vi "数据查询_数据查询.vi"() -> ()   [LabVIEW 2016]
uses:
  <vilib>/Utility/miscctls.llb/LVPointTypeDef.ctl
  <vilib>/Utility/miscctls.llb/LVRowAndColumnUnsignedTypeDef.ctl
  <userlib>/_OpenG.lib/array/array.llb/Sort 2D Array (String)__ogtk.vi
  <vilib>/addons/database/_DB Variant To Data/Database Variant To Data.xnode
panel:
  in  "导出":bool
  out "分钟小时":string(combo)="实时数据"
  out "工作类型":string(combo)="全部数据"
  in  "工作模式":string(combo)="全部数据"
  out "连接的字符串":string
  out "选中数据表":string
  in  "查询":bool
  in  "结束日期":string="2020/01/01"
  in  "起始日期":string="2010/01/01"
  out "XY图":cluster{"data":timestamp[], "data":dbl[]}[](graph)
  in  "组合框":string(combo)
  out "数据表":string[][](table)
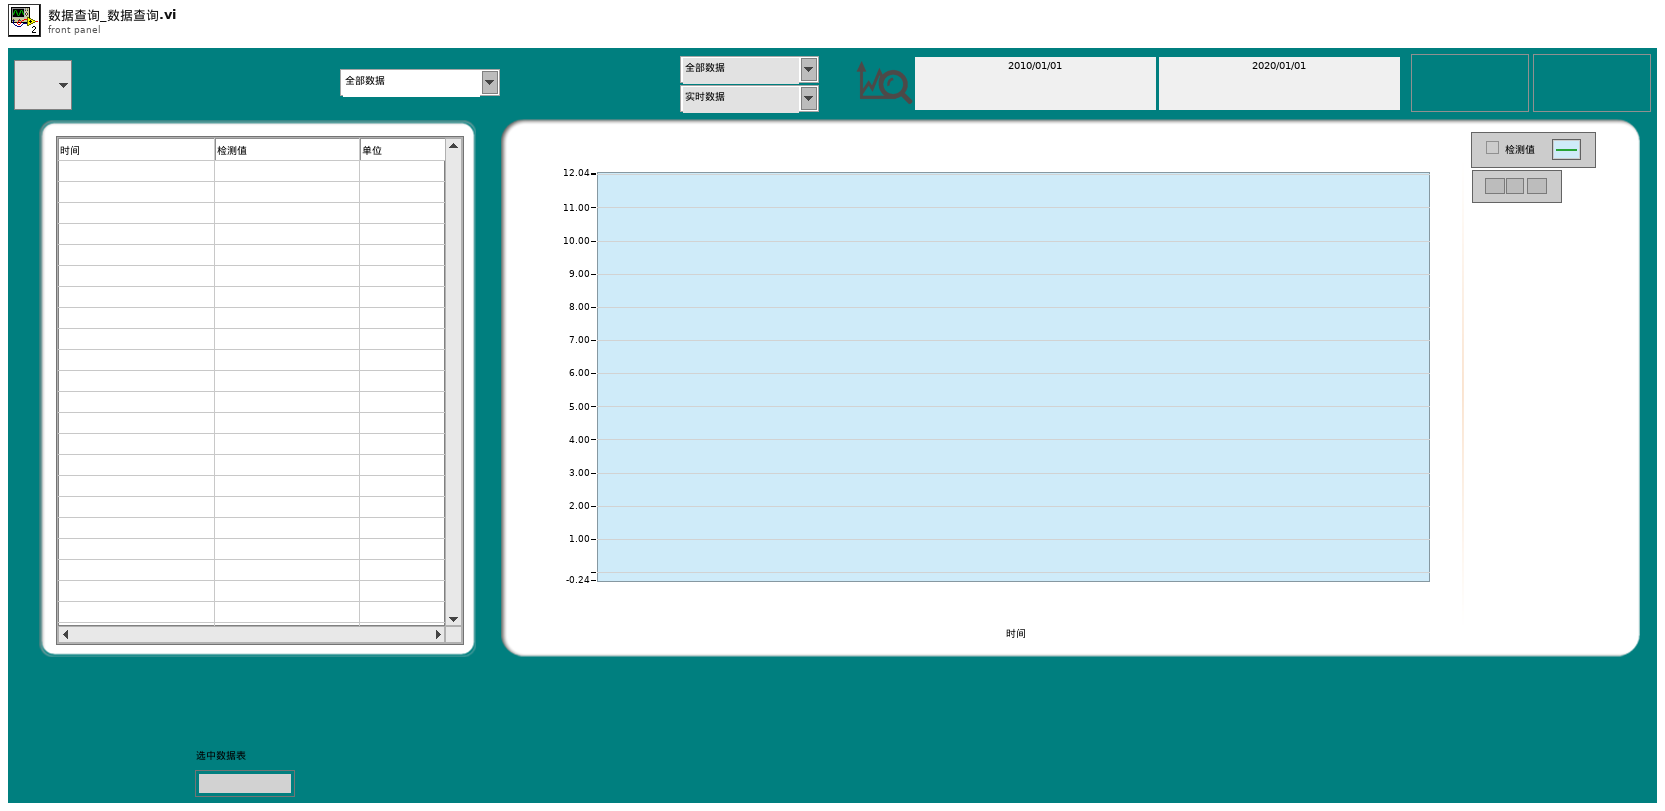
[diagram p1: front panel]
types:
  T1 = typedef "LVPointTypeDef.ctl" = cluster{"Horizontal":i16, "Vertical":i16}
  T2 = enum8{"Enabled", "Disabled", "Disabled and Grayed Out"}
  T3 = typedef "LVRowAndColumnUnsignedTypeDef.ctl" = cluster{"Row":u32, "Column":u32}
  T4 = typedef "LVPoint32TypeDef.ctl" = cluster{"Horizontal":i32, "Vertical":i32}
  T5 = typedef "LVPointDoubleTypeDef.ctl" = cluster{"Cursor X":dbl, "Cursor Y":dbl}
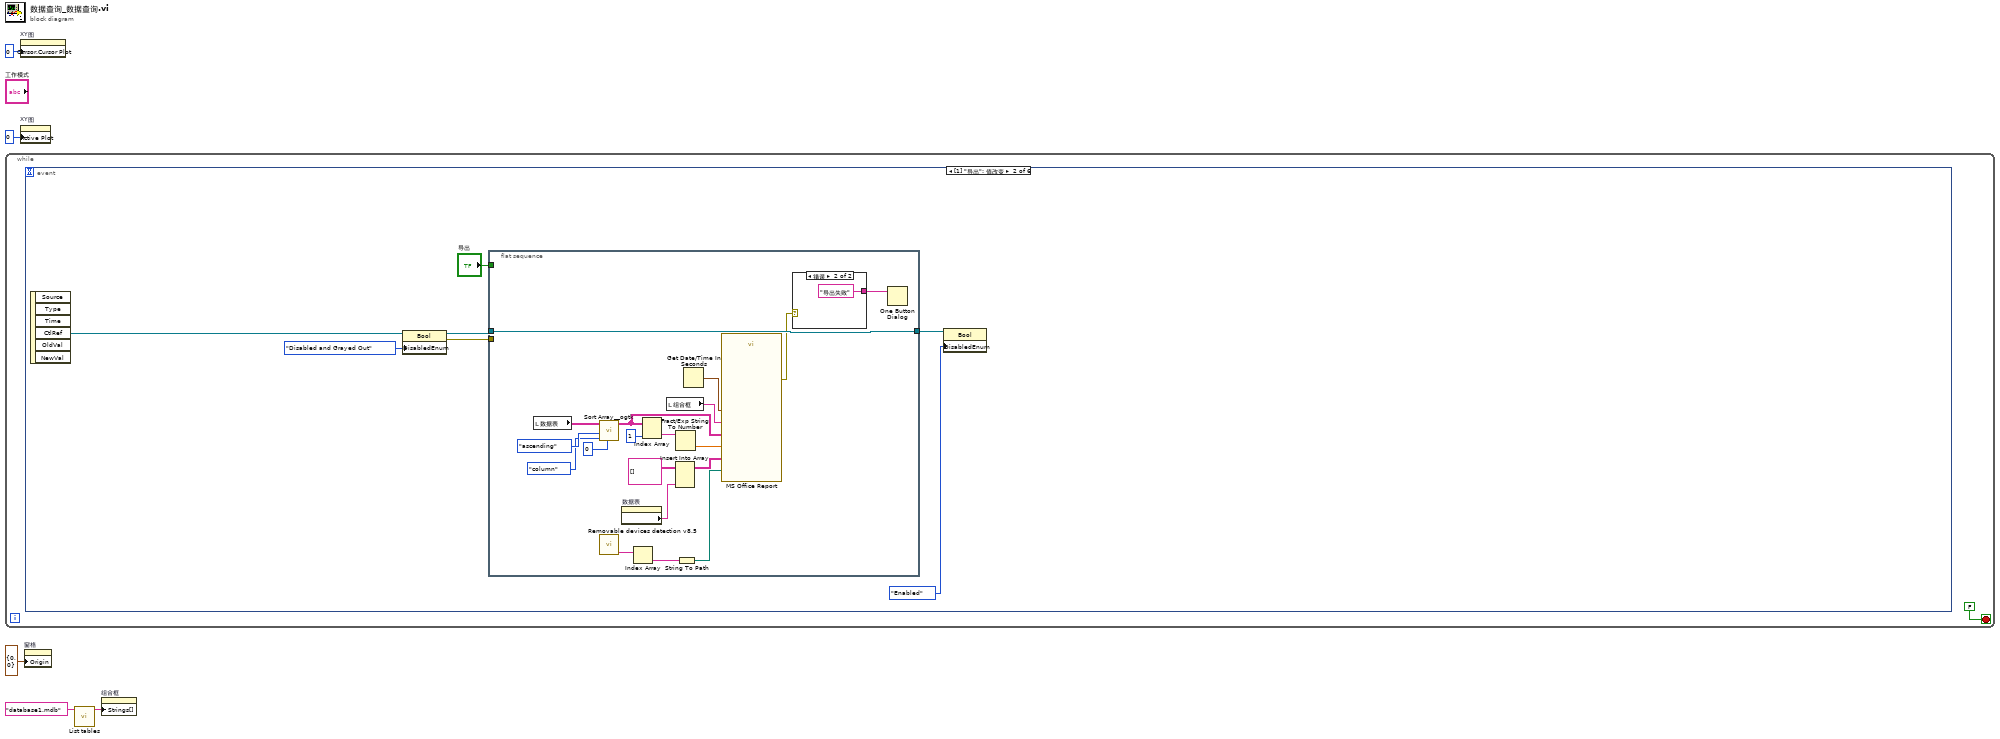
[diagram p0: block diagram]
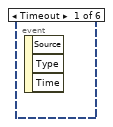
[diagram p2: hidden frame]
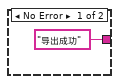
[diagram p3: hidden frame]
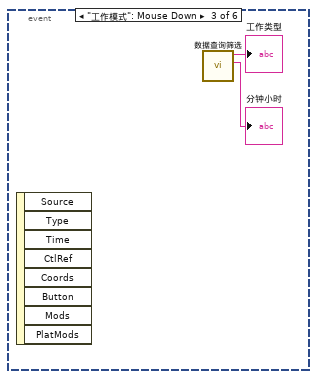
[diagram p4: hidden frame]
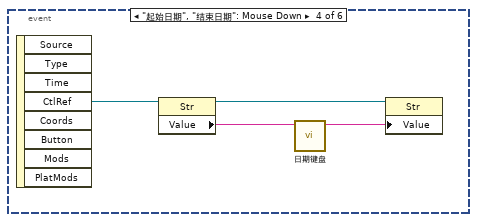
[diagram p5: hidden frame]
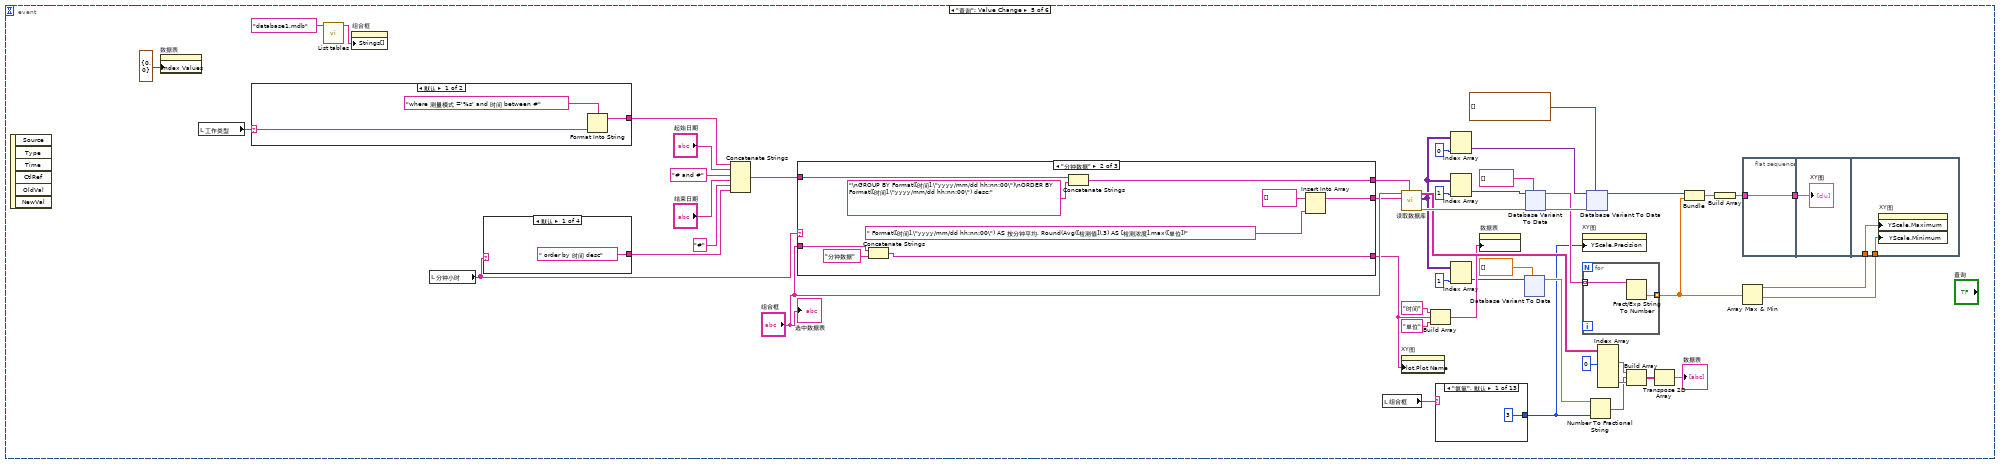
[diagram p6: hidden frame]
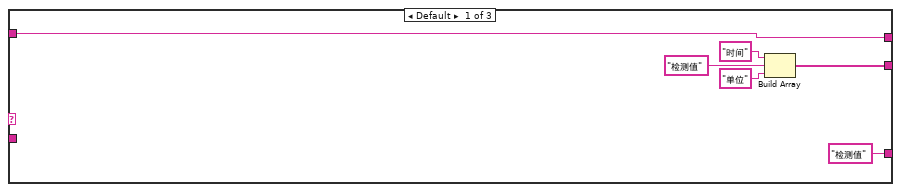
[diagram p7: hidden frame]
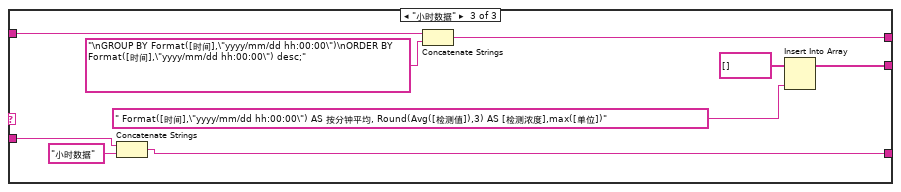
[diagram p8: hidden frame]
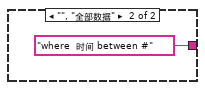
[diagram p12: hidden frame]
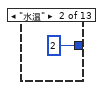
[diagram p13: hidden frame]
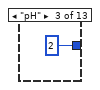
[diagram p14: hidden frame]
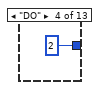
[diagram p15: hidden frame]
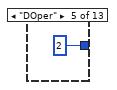
[diagram p16: hidden frame]
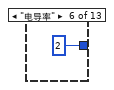
[diagram p17: hidden frame]
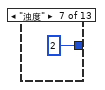
[diagram p18: hidden frame]
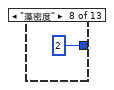
[diagram p19: hidden frame]
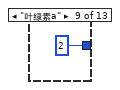
[diagram p20: hidden frame]
diagram:
  n1 = while {
    stop <- FALSE stop-if-true
    n2 = event shown="[1] \"导出\": 值改变" {
      selector: _ -> [_ _ _ _ _ _]
      dyn-events: _ -> [_ _ _ _ _ _]
      timeout: _ -> [_ _ _ _ _ _]
      event Timeout {
        n3 = event-data() -> ()  [unwired: 1 in, 3 out]
      }
      event "导出": Value Change {
        n4 = event-data() -> ("CtlRef"=w13:refnum<vi>)  [unwired: 1 in, 5 out]
        n5 = property class="Bool"(reference=w13, "DisabledEnum"=T2."Disabled and Grayed Out" ("禁用")) -> (reference out=w10:refnum<vi>, error out=w11:errorcluster)  [unwired: 1 in]
        n6 = flat-sequence {
          tunnel: w11 -> [_]
          tunnel: [w22] -> w9
          tunnel: w10 -> [w22]
          tunnel: "导出" -> [_]
          frame #0 {
            n7 = local read "数据表"() -> (w30:string[][])
            n8 = call-poly <userlib>:"Sort Array__ogtk.vi"("Column/Row to Sort By"=u32 0, "Sort By in"=enum16{"row", "column"}."column", "Order"=enum16{"ascending", "descending"}."ascending", "Array in"=w30) -> ("Sorted Array out"=w29:string[][])  [unwired: 4 in, 3 out]
            n9 = call "Removable devices detection v8.5.vi"() -> ("Removable"=w19:string[])  [unwired: 4 out]
            n10 = property on="数据表" class="Tbl (严格)"() -> ("Column Headers[]"=w15:string[])  [unwired: 2 in, 2 out]
            n11 = Index Array(array=w19) -> (element=w18:string)  [unwired: 1 in]
            n12 = Index Array(array=w29, index (col)=1 ("禁用的索引 (列)")) -> (element=w25:string[])  [unwired: 1 in]
            n13 = local read "组合框"() -> (w23:string)
            n14 = Insert Into Array(array=string[][] [], new element=w15) -> (w14:string[][])  [unwired: 2 in]
            n15 = Fract/Exp String To Number(string=w25) -> (number=w24:dbl[])  [unwired: 3 in, 1 out]
            n16 = String To Path(string=w18) -> (path=w17:path)
            n17 = Get Date/Time In Seconds() -> (seconds since 1Jan1904=w32:timestamp)
            n18 = call "MS Office Report"("Path to Save Report"=w17, "导出日期"=w32, "监测参数"=w23, "数据输入"=w29, "图表输入"=w24, "字段定义"=w14) -> ("error out"=w21:errorcluster)  [unwired: 20 in, 1 out]
            n19 = case shown="错误" w21 {
              tunnel: ["导出成功" ("消息") "导出失败" ("消息")] -> w20
              frame No Error {
              }
              frame Error {
              }
            }
            n20 = One Button Dialog(message=w20) -> ()  [unwired: 1 in, 1 out]
          }
        }
        n21 = property class="Bool"(reference=w9, "DisabledEnum"=T2."Enabled" ("禁用")) -> ()  [unwired: 1 in, 2 out]
      }
      event "工作模式": Mouse Down {
        n22 = event-data() -> ()  [unwired: 1 in, 8 out]
        n23 = call "数据查询筛选.vi"() -> ("分钟小时"=→"分钟小时":string, "工作类型"=→"工作类型":string)  [unwired: 10 in]
      }
      event "起始日期", "结束日期": Mouse Down {
        n24 = event-data() -> ("CtlRef"=w40:refnum<vi>)  [unwired: 1 in, 7 out]
        n25 = property class="Str"(reference=w40) -> (reference out=w38:refnum<vi>, "Value"=w39:string)  [unwired: 1 in, 1 out]
        n26 = call "日期键盘.vi"("原值"=w39) -> ("x+y"=w37:string)  [unwired: 10 in]
        n27 = property class="Str"(reference=w38, "Value"=w37) -> ()  [unwired: 1 in, 2 out]
      }
      event "查询": Value Change {
        n28 = event-data() -> ()  [unwired: 1 in, 6 out]
        n29 = property on="数据表" class="Tbl (严格)"("Index Values"=T3 {"Row"=0, "Column"=0} ("索引值")) -> ()  [unwired: 2 in, 2 out]
        n30 = local read "工作类型"() -> (w49:string)
        n31 = case shown="默认" w49 {
          selector: w49 -> [w117 _]
          tunnel: [w115 "where  时间 between #" ("condition")] -> w48
          frame Default {
            n32 = Format Into String(format string="where 测量模式 ='%s' and 时间 between #" ("condition"), w117) -> (resulting string=w115:string)  [unwired: 2 in, 1 out]
          }
          frame "", "全部数据" {
          }
        }
        n33 = call "List tables.vi"("database"="database1.mdb") -> ("tables"=w55:string[])  [unwired: 9 in, 1 out]
        n34 = property on="组合框" class="CmbBox"("Strings[]"=w55) -> ()  [unwired: 2 in, 2 out]
        n35 = local read "分钟小时"() -> (w45:string)
        n36 = case shown="默认" w45 {
          tunnel: [" order by 时间 desc" ("字符串") _ _ _] -> w47
          frame Default {
          }
          frame "分钟数据" {
          }
          frame "小时数据" {
          }
          frame "真" {
          }
        }
        n37 = Concatenate Strings(w48, "起始日期", "# and #" ("condition"), "结束日期", "#" ("condition"), w47) -> (w46:string)
        n38 = case shown="\"分钟数据\"" w45 {
          tunnel: [w91 w103 w108] -> w42
          tunnel: w46 -> [w95 w101 w110]
          tunnel: [w95 w100 w109] -> w44
          tunnel: ["检测值" w96 w105] -> w41
          tunnel: "组合框" -> [_ w97 w107]
          frame Default {
            n39 = Build Array("时间", "检测值", "单位" ("元素")) -> (w91:string[])
          }
          frame "分钟数据" {
            n40 = Concatenate Strings(w97, "分钟数据" ("字符串")) -> (w96:string)
            n41 = Concatenate Strings(w101, "\nGROUP BY Format([时间],\"yyyy/mm/dd hh:nn:00\")\nORDER BY Format([时间],\"yyyy/mm/dd hh:nn:00\") desc;" ("字符串")) -> (w100:string)
            n42 = Insert Into Array(array=string[] [] ("显示项"), new element=" Format([时间],\"yyyy/mm/dd hh:nn:00\") AS 按分钟平均, Round(Avg([检测值]),3) AS [检测浓度],max([单位])" ("新元素/子数组")) -> (w103:string[])  [unwired: 1 in]
          }
          frame "小时数据" {
            n43 = Concatenate Strings(w107, "小时数据" ("字符串")) -> (w105:string)
            n44 = Concatenate Strings(w110, "\nGROUP BY Format([时间],\"yyyy/mm/dd hh:00:00\")\nORDER BY Format([时间],\"yyyy/mm/dd hh:00:00\") desc;" ("字符串")) -> (w109:string)
            n45 = Insert Into Array(array=string[] [] ("显示项"), new element=" Format([时间],\"yyyy/mm/dd hh:00:00\") AS 按分钟平均, Round(Avg([检测值]),3) AS [检测浓度],max([单位])" ("新元素/子数组")) -> (w108:string[])  [unwired: 1 in]
          }
        }
        n46 = local read "组合框"() -> (w56:string)
        n47 = call "读取数据库.vi"("condition"=w44, "显示项"=w42, "组合框"="组合框") -> ("error out"=w80:errorcluster, "data"=w63:variant[][], "表格"=w73:string[][])  [unwired: 5 in, 1 out]
        n48 = property on="XY图" class="XYGraph (严格)"("Plot.Plot Name"=w41) -> ()  [unwired: 2 in, 2 out]
        n49 = Build Array("时间", w41, "单位" ("元素")) -> (w67:string[])
        n50 = case shown="\"氨氮\", 默认" w56 {
          tunnel: [i16 3 ("精度(6)") i16 2 ("精度(6)") i16 2 ("精度(6)") i16 2 ("精度(6)") i16 2 ("精度(6)") i16 2 ("精度(6)") i16 2 ("精度(6)") i16 2 ("精度(6)") i16 2 ("精度(6)") i16 3 ("精度(6)") i16 3 ("精度(6)") i16 2 ("精度(6)") i16 2 ("精度(6)")] -> w50
          frame "氨氮", Default {
          }
          frame "水温" {
          }
          frame "pH" {
          }
          frame "DO" {
          }
          frame "DOper" {
          }
          frame "电导率" {
          }
          frame "浊度" {
          }
          frame "藻密度" {
          }
          frame "叶绿素a" {
          }
          frame "总磷" {
          }
          frame "总氮" {
          }
          frame "CodCr" {
          }
          frame "CodMn" {
          }
        }
        n51 = Index Array(array=w63, index (col)=0 ("禁用的索引 (列)")) -> (element=w83:variant[])  [unwired: 1 in]
        n52 = Index Array(array=w63, index (col)=1 ("禁用的索引 (列)")) -> (element=w81:variant[])  [unwired: 1 in]
        n53 = Index Array(array=w63, index (col)=1 ("禁用的索引 (列)")) -> (element=w61:variant[])  [unwired: 1 in]
        n54 = property on="数据表" class="Tbl (严格)"("Column Headers[]"=w67) -> ()  [unwired: 2 in, 2 out]
        n55 = xnode "Database Variant To Data"("database variant"=w61, "type"=sgl[] []) -> ("data"=w59:sgl[])  [unwired: 1 in, 1 out]
        n56 = xnode "Database Variant To Data"("database variant"=w81, "error in (no error)"=w80, "type"=string[] []) -> ("data"=w66:string[], "error out"=w79:errorcluster)
        n57 = property on="XY图" class="XYGraph (严格)"("YScale.Precision"=w50) -> ()  [unwired: 2 in, 2 out]
        n58 = for {
          tunnel: w66 -> [w171] mode=indexing
          tunnel: [w170] -> w53 mode=indexing
          n59 = Fract/Exp String To Number(string=w171) -> (number=w170:dbl)  [unwired: 3 in, 1 out]
        }
        n60 = xnode "Database Variant To Data"("database variant"=w83, "error in (no error)"=w79, "type"=timestamp[] []) -> ("data"=w74:timestamp[])  [unwired: 1 out]
        n61 = Number To Fractional String(number=w59, precision (6)=w50) -> (F-format string=w58:string[])  [unwired: 2 in]
        n62 = Index Array(array=w73, index (col) #1=0 ("禁用的索引 (列)")) -> (element #1=w71:string[], element #3=w64:string[])  [unwired: 5 in, 1 out]
        n63 = Build Array(w71, w58, w64) -> (w70:string[][])
        n64 = Transpose 2D Array(2D array=w70) -> (transposed array=→"数据表":string[][])
        n65 = Bundle("data"=w74, w53) -> (w75:cluster{"data":timestamp[], dbl[]})  [unwired: 1 in]
        n66 = Build Array(w75) -> (w76:cluster{"data":timestamp[], dbl[]}[])
        n67 = flat-sequence {
          tunnel: [w172] -> w77
          tunnel: w76 -> [w172]
          tunnel: w77 -> [w173]
          tunnel: w52 -> [w175]
          tunnel: w51 -> [w174]
          frame #0 {
          }
          frame #1 {
            "XY图" <- w173
          }
          frame #2 {
            n68 = property on="XY图" class="XYGraph (严格)"("YScale.Maximum"=w175, "YScale.Minimum"=w174) -> ()  [unwired: 2 in, 2 out]
          }
        }
        n69 = Array Max & Min(array=w53) -> (max value=w52:dbl, min value=w51:dbl)  [unwired: 2 out]
        "选中数据表" <- "组合框"
      }
      event "XY图": Mouse Move {
        w270 = "   " ("字符串")
        n70 = event-data() -> ("CtlRef"=w280:refnum<vi>, "Coords"=w279:T4)  [unwired: 1 in, 3 out]
        n71 = invoke class="XYGraph (严格)" method="Map Coords To XY"(reference=w280, "Coords"=w279) -> (reference out=w278:refnum<vi>, error out=w275:errorcluster, "XY"=w277:cluster{"X":dbl, "Y":dbl})  [unwired: 5 in, 4 out]
        n72 = property class="XYGraph (严格)"(reference=w278, error in=w275, "Cursor.Cursor Position"=w277) -> (error out=w276:errorcluster)  [unwired: 1 out]
        n73 = property on="XY图" class="XYGraph (严格)"(error in=w276) -> ("Cursor.Cursor Position"=w273:T5, "YScale.Precision"=w266:u8)  [unwired: 1 in, 2 out]
        n74 = Unbundle(w273) -> ("Cursor X"=w272:dbl, "Cursor Y"=w269:dbl)
        n75 = property on="XY图" class="XYGraph (严格)"() -> ("Plot.Plot Name"=w267:string)  [unwired: 2 in, 2 out]
        n76 = Number To Fractional String(number=w269, precision (6)=w266) -> (F-format string=w268:string)  [unwired: 2 in]
        n77 = Format Date/Time String(seconds (now)=w272) -> (date/time string=w271:string)  [unwired: 2 in]
        n78 = Concatenate Strings(w267, w270, w271, w270, w268) -> (→"连接的字符串":string)
      }
    }
  }
  n79 = property on="XY图" class="XYGraph (严格)"("Cursor.Cursor Plot"=0 ("游标.游标关联曲线")) -> ()  [unwired: 2 in, 2 out]
  n80 = property on="XY图" class="XYGraph (严格)"("Active Plot"=u32 0 ("活动曲线")) -> ()  [unwired: 2 in, 2 out]
  n81 = property on="窗格" class="Pane"("Origin"=T1 {"Horizontal"=0, "Vertical"=0} ("原点")) -> ()  [unwired: 2 in, 2 out]
  n82 = call "List tables.vi"("database"="database1.mdb") -> ("tables"=w1:string[])  [unwired: 9 in, 1 out]
  n83 = property on="组合框" class="CmbBox"("Strings[]"=w1) -> ()  [unwired: 2 in, 2 out]
